vi "Update Line.vi"(0 "Display State In":T1={"logTable"=refnum, "max items"=500, "displaydata"=[], "data"=[], "Auto Scroll"=TRUE, "current item"=500, "col headers"=[], "Add to Top"=TRUE, "Auto resize"=TRUE, "col size"=[], "filters"=[], "color cells"=[]}, 5 "Line":string[](array[string]), 7 "column":string, 9 "Container State":T3, 11 "error in (no error)":errorcluster) -> (4 "Display State Out":T1={"logTable"=refnum, "max items"=500, "displaydata"=[], "data"=[], "Auto Scroll"=TRUE, "current item"=500, "col headers"=[], "Add to Top"=TRUE, "Auto resize"=TRUE, "col size"=[], "filters"=[], "color cells"=[]}, 15 "error out":errorcluster)   [LabVIEW 2013, in "UI-DisplayTable(dev).xctl"]
uses:
  UI-DisplayTable(dev).xctl
  <vilib>/_xctls/Container State.ctl
  State.ctl
  Support/DEF-Filter.ctl
  <vilib>/_xctls/XControlSupport.lvlib
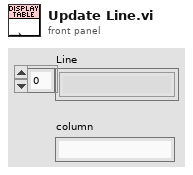
[diagram p1: front panel]
types:
  T1 = typedef "UI-DisplayTable(dev).xctl/State.ctl" = cluster{"logTable":refnum<vi>, "max items":i32, "displaydata":string[][], "data":string[][], "Auto Scroll":bool, "current item":i32, "col headers":string[], "Add to Top":bool, "Auto resize":bool, "col size":i32[], "filters":T2[], "color cells":cluster{"color cell":cluster{"Column":string, "Value":string, "Highlight Column":string}, "Color Box":u32}[]}
  T2 = typedef "UI-DisplayTable(dev).xctl/DEF-Filter.ctl" = cluster{"column":string, "value":string[]}
  T3 = typedef "XControlSupport.lvlib/Container State.ctl" = cluster{"Indicator?":bool, "Run Mode?":bool, " Refnum":refnum<vi>}
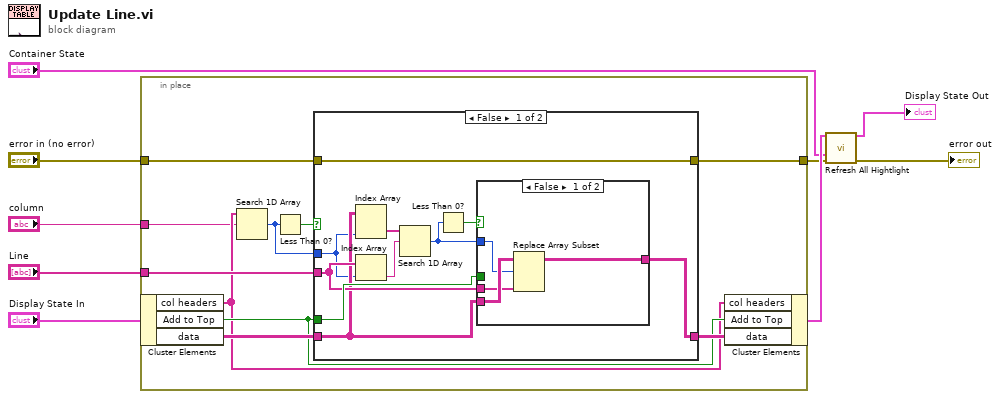
[diagram p0: block diagram]
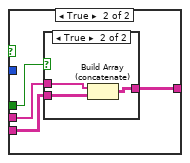
[diagram p2: hidden frame]
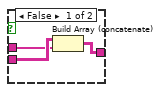
[diagram p3: hidden frame]
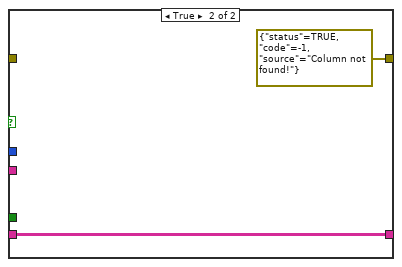
[diagram p4: hidden frame]
diagram:
  n1 = in-place {
    in-place-border: "Line" -> [w18]
    in-place-border: "column" -> [w14]
    in-place-border: [w13] -> w3
    in-place-border: "error in (no error)" -> [w12]
    n2 = in-place-cluster #1("Display State In") -> ("col headers"=w15:string[], "Add to Top"=w16:bool, "data"=w19:string[][])
    n3 = Search 1D Array(1D array=w15, element=w14) -> (index of element=w10:i32)  [unwired: 1 in]
    n4 = Less Than 0?(x=w10) -> (x < 0?=w11:bool)
    n5 = case shown="False" w11 {
      tunnel: w19 -> [w25 w44]
      tunnel: w18 -> [w26 _]
      tunnel: [w29 w44] -> w17
      tunnel: w16 -> [w28 _]
      tunnel: [w27 errorcluster {"status"=TRUE, "code"=-1, "source"="Column not found!"} ("error in (no error)")] -> w13
      tunnel: w12 -> [w27 _]
      tunnel: w10 -> [w24 _]
      frame False {
        n6 = Index Array(array=w25, index (col)=w24) -> (element=w23:string[])  [unwired: 1 in]
        n7 = Index Array(array=w26, index=w24) -> (element=w22:string)
        n8 = Search 1D Array(1D array=w23, element=w22) -> (index of element=w20:i32)  [unwired: 1 in]
        n9 = Less Than 0?(x=w20) -> (x < 0?=w21:bool)
        n10 = case shown="False" w21 {
          tunnel: [w31 w37] -> w29
          tunnel: w28 -> [_ w36]
          tunnel: w26 -> [w32 w35]
          tunnel: w25 -> [w33 w34]
          tunnel: w20 -> [w30 _]
          frame False {
            n11 = Replace Array Subset(array=w33, new element=w32, index (row)=w30) -> (w31:string[][])  [unwired: 1 in]
          }
          frame True {
            n12 = case shown="True" w36 {
              tunnel: w34 -> [w40 w43]
              tunnel: w35 -> [w39 w41]
              tunnel: [w38 w42] -> w37
              frame False {
                n13 = Build Array (concatenate)(w40, w39) -> (w38:string[][])
              }
              frame True {
                n14 = Build Array (concatenate)(w41, w43) -> (w42:string[][])
              }
            }
          }
        }
      }
      frame True {
      }
    }
    n15 = in-place-cluster #1("col headers"=w15, "Add to Top"=w16, "data"=w17) -> (w5:T1)
  }
  n16 = call "Refresh All Hightlight.vi"("Display State In"=w5, "Container State"="Container State", "error in (no error)"=w3) -> ("Display State Out"=→"Display State Out":T1, "error out"=→"error out":errorcluster)  [unwired: 11 in]
